vi "Configure Channel.vi"(0 "VISA resource name":refnum<visa-resource-name>, 1 "Enable Channel (T:Enable)":bool=TRUE, 5 "Channel (1: Channel 1)":u16(ring)=1 items=["Channel 1"=1, "Channel 2"=2], 7 "Vertical Coupling (1: DC)":u16(ring)=1 items=["AC", "DC", "Ground"], 9 "Probe Attenuation (1.0)":dbl=1.0, 11 "error in (no error)":errorcluster, 12 "Vertical Range (10.0 V)":dbl=10.0, 13 "Vertical Offset (0.0 V)":dbl) -> (4 "VISA resource name out":refnum<visa-resource-name>, 15 "error out":errorcluster)   [LabVIEW 2020, in "Template - Scope.lvlib"]
doc: "Configures the common properties of the vertical subsystem of the oscilloscope for the specified channel. Call this VI for each channel you want to enable to acquire waveforms.\n\n<B>Note:</B>\nThe channel settings will not be applied if the channel is not enabled."
uses:
  <instrlib>/_Template - Scope/Template - Scope.lvlib
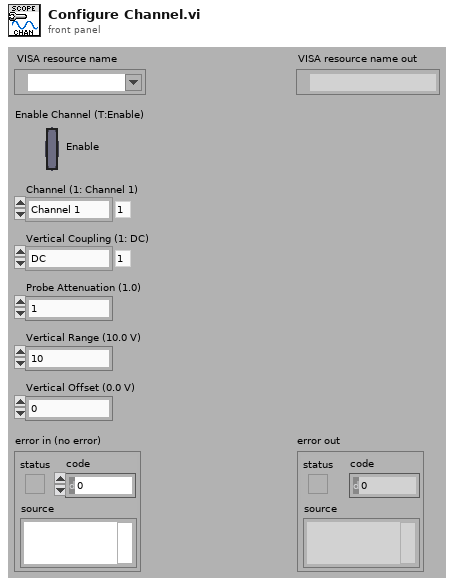
[diagram p1: front panel]
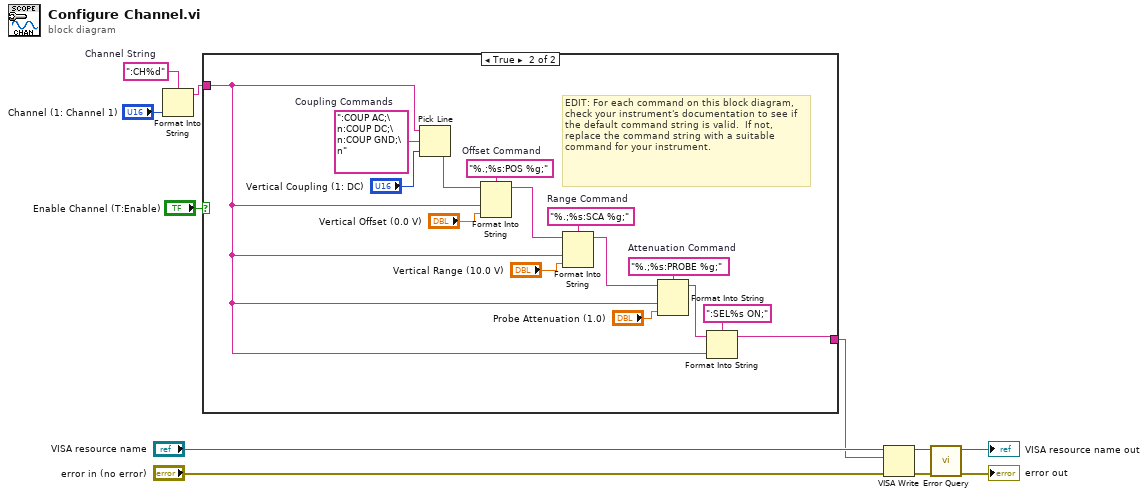
[diagram p0: block diagram]
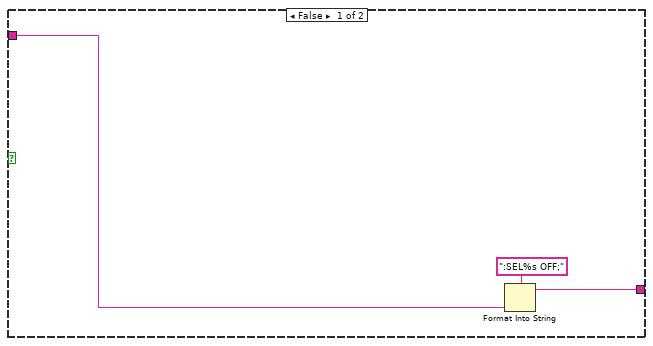
[diagram p2: hidden frame]
diagram:
  w2 = ":CH%d"  # Channel String
  n1 = Format Into String(format string=w2, "Channel (1: Channel 1)") -> (resulting string=w1:string)  [unwired: 2 in, 1 out]
  n2 = case shown="True" "Enable Channel (T:Enable)" {
    tunnel: [w12 w18] -> w5
    tunnel: w1 -> [w13 w15]
    frame False {
      n3 = Format Into String(format string=":SEL%s OFF;", w13) -> (resulting string=w12:string)  [unwired: 2 in, 1 out]
    }
    frame True {
      w24 = "%.;%s:PROBE %g;"  # Attenuation Command
      w25 = "%.;%s:SCA %g;"  # Range Command
      w27 = "%.;%s:POS %g;"  # Offset Command
      w29 = ":COUP AC;\n:COUP DC;\n:COUP GND;\n"  # Coupling Commands
      # "EDIT: For each command on this block diagram, check your instrument's documentation to see if the default command string is valid.  If not, replace the command string with a suitable command for your instrument."
      n4 = Pick Line(string ("")=w15, multi-line string=w29, line index="Vertical Coupling (1: DC)") -> (output string=w17:string)
      n5 = Format Into String(format string=w27, initial string=w17, w15, "Vertical Offset (0.0 V)") -> (resulting string=w16:string)  [unwired: 1 in, 1 out]
      n6 = Format Into String(format string=w25, initial string=w16, w15, "Vertical Range (10.0 V)") -> (resulting string=w21:string)  [unwired: 1 in, 1 out]
      n7 = Format Into String(format string=w24, initial string=w21, w15, "Probe Attenuation (1.0)") -> (resulting string=w19:string)  [unwired: 1 in, 1 out]
      n8 = Format Into String(format string=":SEL%s ON;", initial string=w19, w15) -> (resulting string=w18:string)  [unwired: 1 in, 1 out]
    }
  }
  n9 = VISA Write(VISA resource name="VISA resource name", write buffer=w5, error in (no error)="error in (no error)") -> (VISA resource name out=w7:refnum<visa-resource-name>, error out=w6:errorcluster)  [unwired: 1 out]
  n10 = call <instrlib>:"Error Query.vi"("error in (no error)"=w6, "VISA resource name"=w7) -> ("error out"=→"error out":errorcluster, "VISA resource name out"=→"VISA resource name out":refnum<visa-resource-name>)  [unwired: 6 in, 2 out]
